vi "Compile - Rx Packet Information.vi"(8 "error in (no error)":errorcluster, 11 "Custom Device Ref in":T1 format="%.0x") -> (0 "error out":errorcluster, 1 "Rx Ref Array":T2(array[cluster]) {"VS Refs" format="%.0x"}, 2 "Rx Packet Info Array":T3[](array[typedef]) {"Endianness" items=["big-endian"=0, "little-indian"=2]}, 3 "Custom Device Ref out":T1 format="%.0x")   [LabVIEW 2016, in "UDP-Custom-Device System Explorer.lvlib"]
uses:
  UDP-Custom-Device System Explorer.lvlib
  Shared/Types/Shared - Rx.PacketInfo.ctl
  Shared/Types/Shared - Channel Data Type.ctl
  Shared/Types/Shared - Buffered.PacketInfo.ctl
  Shared/Types/Shared - Pointer Encoding.ctl
  Shared/Types/Shared - Buffer Options.ctl
  Shared/Types/Shared - Duplex Settings.ctl
  Shared/Types/Shared - New Data Options.ctl
  <vilib>/NI Veristand/Custom Device API/Custom Device Item Ref.ctl
  Shared/UDP-Custom-Device Shared.lvlib
  <vilib>/NI VeriStand/Custom Device API/Custom Device API.lvlib
  Property Accessors/Rx Channel Accessors.lvlib
  Property Accessors/Shared Packet Accessors.lvlib
  Property Accessors/Rx Packet Accessors.lvlib
  Property Accessors/Buffered Data Packet.lvlib
  Property Accessors/Rx Channel Section Accessors.lvlib
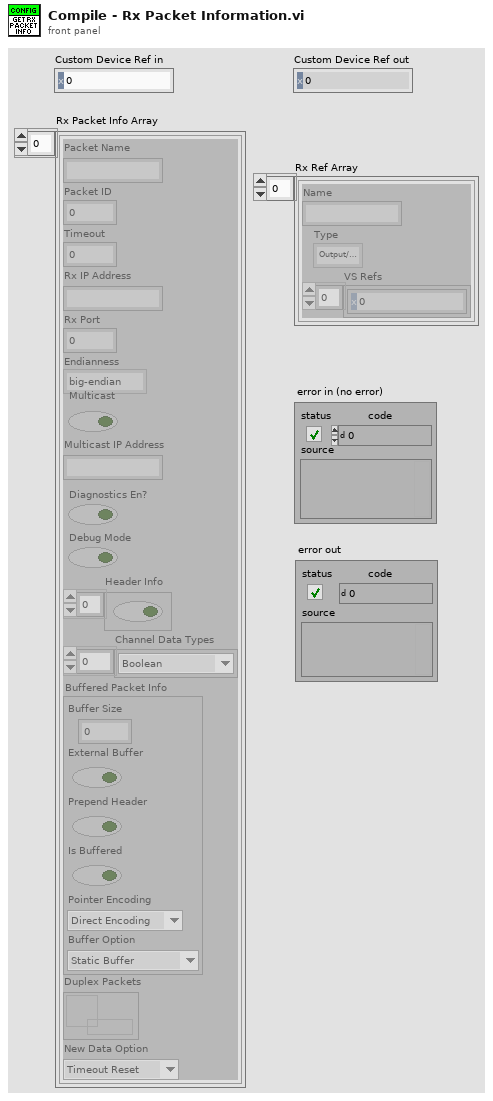
[diagram p1: front panel]
types:
  T1 = typedef "Custom Device API.lvlib/Custom Device Item Ref.ctl" = u64
  T2 = cluster{"Name":string, "Type":enum16{"Output/Write", "Input/Read", "Input/ReadWrite"}, "VS Refs":T1[]}[]
  T3 = typedef "UDP-Custom-Device Shared.lvlib/Shared - Rx.PacketInfo.ctl" = cluster{"Packet Name":string, "Packet ID":i32, "Timeout":i32, "Rx IP Address":string, "Rx Port":u16, "Endianness":u16, "Multicast":bool, "Multicast IP Address":string, "Diagnostics En?":bool, "Debug Mode":bool, "Header Info":bool[], "Channel Data Types":T4[], "Buffered Packet Info":T5, "Duplex Packets":refnum<data-value>, "New Data Option":T8}
  T4 = typedef "UDP-Custom-Device Shared.lvlib/Shared - Channel Data Type.ctl" = enum16{"Boolean", "Single", "Double", "I8", "I16", "I32", "I64", "U8", "U16", "U32", "U64"}
  T5 = typedef "UDP-Custom-Device Shared.lvlib/Shared - Buffered.PacketInfo.ctl" = cluster{"Buffer Size":i32, "External Buffer":bool, "Prepend Header":bool, "Is Buffered":bool, "Pointer Encoding":T6, "Buffer Option":T7}
  T6 = typedef "UDP-Custom-Device Shared.lvlib/Shared - Pointer Encoding.ctl" = enum16{"Direct Encoding", "Conversion Encoding"}
  T7 = typedef "UDP-Custom-Device Shared.lvlib/Shared - Buffer Options.ctl" = enum16{"Static Buffer", "Circular Buffer"}
  T8 = typedef "UDP-Custom-Device Shared.lvlib/Shared - New Data Options.ctl" = enum16{"Timeout Reset", "Counter"}
  T9 = typedef "UDP-Custom-Device System Explorer.lvlib/Packet Type.ctl" = enum16{"Transmit", "Receive", "Buffered Transmit", "Buffered Receive"}
  T10 = typedef "Custom Device API.lvlib/Custom Device Item Info.ctl" = cluster{"Name":string, "Is Channel":bool, "GUID":string, "Is Waveform":bool}
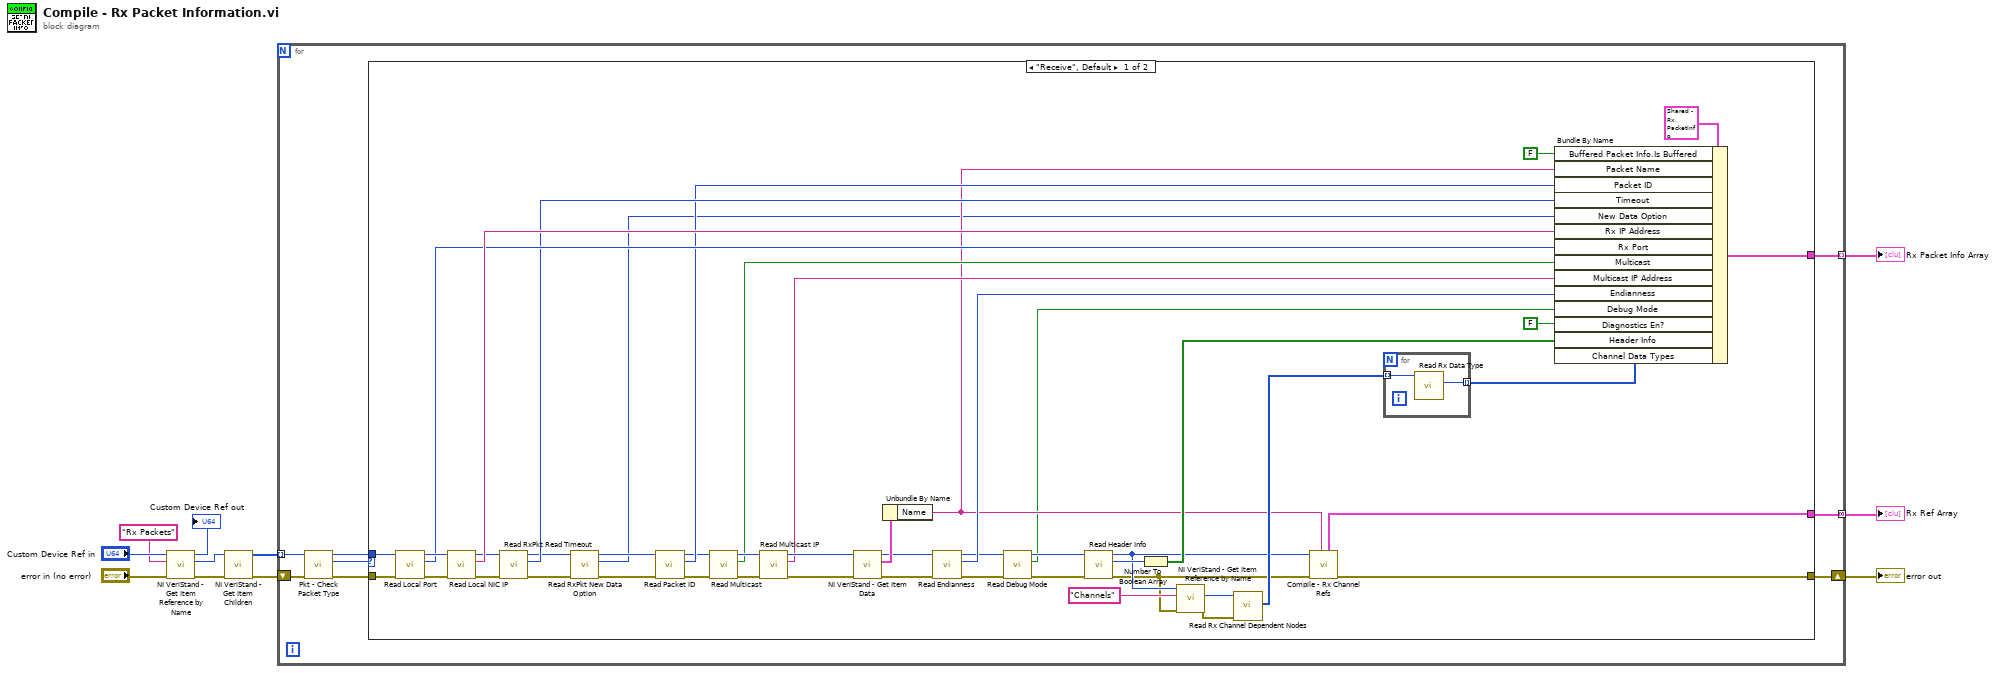
[diagram p0: block diagram]
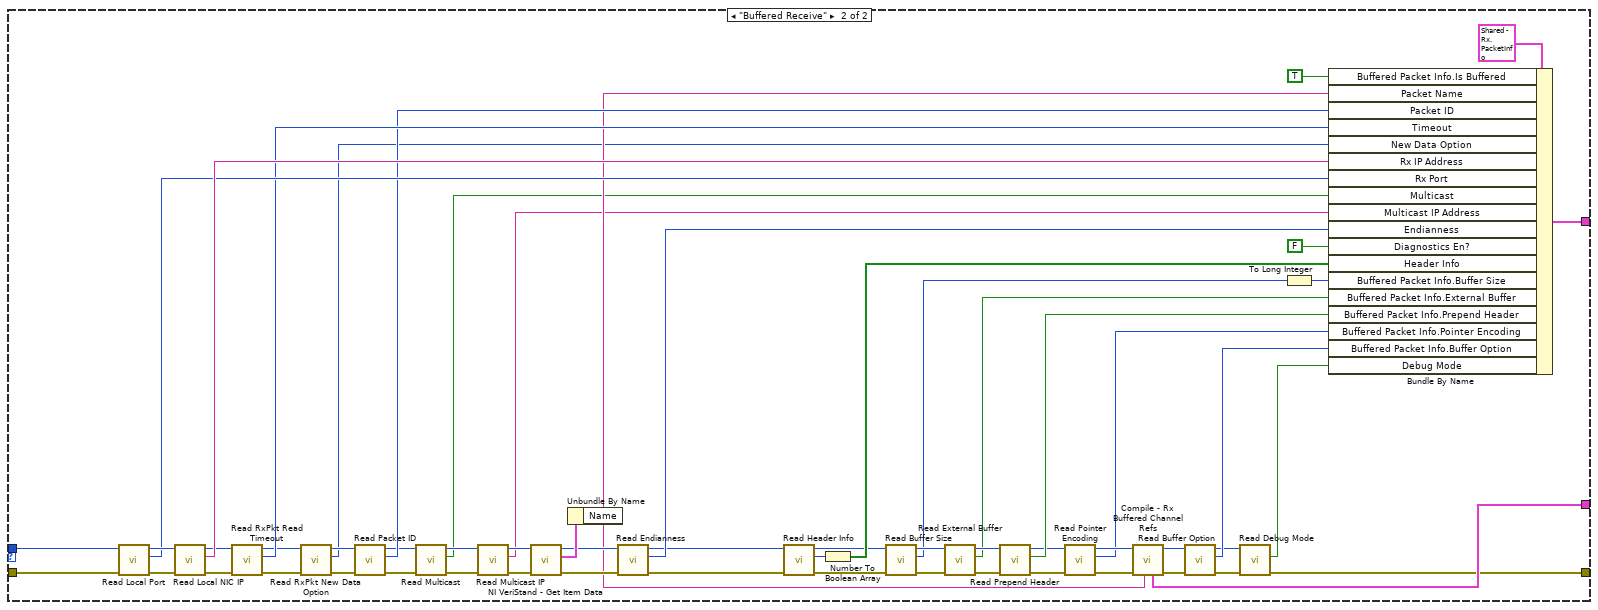
[diagram p2: hidden frame]
diagram:
  n1 = call <vilib>:"NI VeriStand - Get Item Reference by Name.vi"("error in (no error)"="error in (no error)", "Item Name"="Rx Packets", "Parent Ref in"="Custom Device Ref in") -> ("error out"=w5:errorcluster, "Item Ref"=w2:T1, "Parent Ref out"=→"Custom Device Ref out":T1)  [unwired: 5 in, 1 out]
  n2 = call <vilib>:"NI VeriStand - Get Item Children.vi"("error in (no error)"=w5, "Item Ref in"=w2) -> ("error out"=w8:errorcluster, "Child Refs"=w7:T1[])  [unwired: 6 in, 2 out]
  n3 = for {
    tunnel: w7 -> [w17] mode=indexing
    shift-right: [w18] -> w10
    shift-left: w8 -> [w15]
    tunnel: [w19] -> w9 mode=indexing
    tunnel: [w13] -> w6 mode=concatenating
    n4 = call "Pkt - Check Packet Type.vi"("error in (no error)"=w15, "Node Ptr In"=w17) -> ("error out"=w14:errorcluster, "Packet Type"=w12:T9, "Node Ptr Out"=w16:T1)  [unwired: 7 in]
    n5 = case shown="\"Receive\", Default" w12 {
      tunnel: [w66 w127] -> w19
      tunnel: [w32 w71] -> w18
      tunnel: w16 -> [w45 w110]
      tunnel: w14 -> [w44 w109]
      tunnel: [w31 w95] -> w13
      frame "Receive", Default {
        n6 = call "Read Local Port.vi"("error in (no error)"=w44, "Node Ptr"=w45) -> ("error out"=w56:errorcluster, "Port"=w57:u16, "Node Ptr out"=w59:T1)  [unwired: 7 in]
        n7 = call "Read Local NIC IP.vi"("error in (no error)"=w56, "Node Ptr"=w59) -> ("error out"=w52:errorcluster, "IP Address of Local NIC"=w58:string, "Node Ptr out"=w53:T1)  [unwired: 7 in]
        n8 = call "Read RxPkt Read Timeout.vi"("error in (no error)"=w52, "Node Ptr"=w53) -> ("error out"=w27:errorcluster, "Read Timeout"=w55:i32, "Node Ptr out"=w29:T1)  [unwired: 7 in]
        n9 = call "Read RxPkt New Data Option.vi"("error in (no error)"=w27, "Node Ptr"=w29) -> ("error out"=w26:errorcluster, "New Data Option"=w25:T8, "Node Ptr out"=w28:T1)  [unwired: 7 in]
        n10 = call "Read Packet ID.vi"("error in (no error)"=w26, "Node Ptr"=w28) -> ("error out"=w36:errorcluster, "Packet ID"=w54:i32, "Node Ptr out"=w35:T1)  [unwired: 7 in]
        n11 = call "Read Multicast.vi"("error in (no error)"=w36, "Node Ptr"=w35) -> ("error out"=w41:errorcluster, "Multicast"=w38:bool, "Node Ptr out"=w42:T1)  [unwired: 7 in]
        n12 = call "Read Multicast IP.vi"("error in (no error)"=w41, "Node Ptr"=w42) -> ("error out"=w39:errorcluster, "Multicast IP Address"=w37:string, "Node Ptr out"=w40:T1)  [unwired: 7 in]
        n13 = call <vilib>:"NI VeriStand - Get Item Data.vi"("error in (no error)"=w39, "Item Ref in"=w40) -> ("error out"=w48:errorcluster, "Item Info"=w51:T10, "Item Ref out"=w49:T1)  [unwired: 6 in, 1 out]
        n14 = Unbundle By Name(w51) -> ("Name"=w30:string)
        n15 = call "Read Endianness.vi"("error in (no error)"=w48, "Node Ptr"=w49) -> ("error out"=w22:errorcluster, "Endianness"=w47:u16, "Node Ptr out"=w24:T1)  [unwired: 7 in]
        n16 = call "Read Debug Mode.vi"("error in (no error)"=w22, "Node Ptr"=w24) -> ("error out"=w21:errorcluster, "Debug Mode"=w20:bool, "Node Ptr out"=w23:T1)  [unwired: 7 in]
        n17 = call "Read Header Info.vi"("error in (no error)"=w21, "Node Ptr"=w23) -> ("error out"=w33:errorcluster, "Header Info"=w46:u32, "Node Ptr out"=w34:T1)  [unwired: 7 in]
        n18 = Number To Boolean Array(number=w46) -> (Boolean array=w65:bool[])
        n19 = call <vilib>:"NI VeriStand - Get Item Reference by Name.vi"("error in (no error)"=w33, "Item Name"="Channels" ("Section Name"), "Parent Ref in"=w34) -> ("error out"=w62:errorcluster, "Item Ref"=w63:T1)  [unwired: 5 in, 2 out]
        n20 = call "Read Rx Channel Dependent Nodes.vi"("error in (no error)"=w62, "Node Ptr"=w63) -> ("Dependent Node Refs"=w61:T1[])  [unwired: 7 in, 2 out]
        n21 = call "Compile - Rx Channel Refs.vi"("Packet Name"=w30, "error in (no error)"=w33, "Item Ref in"=w34) -> ("error out"=w32:errorcluster, "Rx Ref Array"=w31:T2)  [unwired: 6 in, 1 out]
        n22 = for {
          tunnel: w61 -> [w69] mode=indexing
          tunnel: [w68] -> w60 mode=indexing
          n23 = call "Read Rx Data Type.vi"("Node Ptr"=w69) -> ("Data Type"=w68:T4)  [unwired: 8 in, 2 out]
        }
        n24 = Bundle By Name(cluster=T3 {"Packet Name"="", "Packet ID"=0, "Timeout"=0, "Rx IP Address"="", "Rx Port"=0, "Endianness"=0, "Multicast"=FALSE, "Multicast IP Address"="", "Diagnostics En?"=FALSE, "Debug Mode"=FALSE, "Header Info"=[], "Channel Data Types"=[], "Buffered Packet Info"={"Buffer Size"=0, "External Buffer"=FALSE, "Prepend Header"=FALSE, "Is Buffered"=FALSE, "Pointer Encoding"=enum."Direct Encoding", "Buffer Option"=enum."Static Buffer"}, "Duplex Packets"=refnum, "New Data Option"=enum."Timeout Reset"} ("Packet Info"), "Buffered Packet Info.Is Buffered"=FALSE, "Packet Name"=w30, "Packet ID"=w54, "Timeout"=w55, "New Data Option"=w25, "Rx IP Address"=w58, "Rx Port"=w57, "Multicast"=w38, "Multicast IP Address"=w37, "Endianness"=w47, "Debug Mode"=w20, "Diagnostics En?"=FALSE, "Header Info"=w65, "Channel Data Types"=w60) -> (w66:T3)
      }
      frame "Buffered Receive" {
        n25 = call "Read Local Port.vi"("error in (no error)"=w109, "Node Ptr"=w110) -> ("error out"=w123:errorcluster, "Port"=w124:u16, "Node Ptr out"=w126:T1)  [unwired: 7 in]
        n26 = call "Read Local NIC IP.vi"("error in (no error)"=w123, "Node Ptr"=w126) -> ("error out"=w119:errorcluster, "IP Address of Local NIC"=w125:string, "Node Ptr out"=w120:T1)  [unwired: 7 in]
        n27 = call "Read RxPkt Read Timeout.vi"("error in (no error)"=w119, "Node Ptr"=w120) -> ("error out"=w81:errorcluster, "Read Timeout"=w122:i32, "Node Ptr out"=w79:T1)  [unwired: 7 in]
        n28 = call "Read RxPkt New Data Option.vi"("error in (no error)"=w81, "Node Ptr"=w79) -> ("error out"=w80:errorcluster, "New Data Option"=w77:T8, "Node Ptr out"=w78:T1)  [unwired: 7 in]
        n29 = call "Read Packet ID.vi"("error in (no error)"=w80, "Node Ptr"=w78) -> ("error out"=w87:errorcluster, "Packet ID"=w121:i32, "Node Ptr out"=w88:T1)  [unwired: 7 in]
        n30 = call "Read Multicast.vi"("error in (no error)"=w87, "Node Ptr"=w88) -> ("error out"=w93:errorcluster, "Multicast"=w90:bool, "Node Ptr out"=w94:T1)  [unwired: 7 in]
        n31 = call "Read Multicast IP.vi"("error in (no error)"=w93, "Node Ptr"=w94) -> ("error out"=w92:errorcluster, "Multicast IP Address"=w89:string, "Node Ptr out"=w91:T1)  [unwired: 7 in]
        n32 = call <vilib>:"NI VeriStand - Get Item Data.vi"("error in (no error)"=w92, "Item Ref in"=w91) -> ("error out"=w115:errorcluster, "Item Info"=w118:T10, "Item Ref out"=w116:T1)  [unwired: 6 in, 1 out]
        n33 = Unbundle By Name(w118) -> ("Name"=w96:string)
        n34 = call "Read Endianness.vi"("error in (no error)"=w115, "Node Ptr"=w116) -> ("error out"=w112:errorcluster, "Endianness"=w114:u16, "Node Ptr out"=w113:T1)  [unwired: 7 in]
        n35 = call "Read Header Info.vi"("error in (no error)"=w112, "Node Ptr"=w113) -> ("error out"=w98:errorcluster, "Header Info"=w111:u32, "Node Ptr out"=w99:T1)  [unwired: 7 in]
        n36 = Number To Boolean Array(number=w111) -> (Boolean array=w107:bool[])
        n37 = call "Read Buffer Size.vi"("error in (no error)"=w98, "Node Ptr"=w99) -> ("error out"=w106:errorcluster, "Buffer Size"=w103:u32, "Node Ptr out"=w104:T1)  [unwired: 7 in]
        n38 = call "Read External Buffer.vi"("error in (no error)"=w106, "Node Ptr"=w104) -> ("error out"=w105:errorcluster, "External Buffer"=w97:bool, "Node Ptr out"=w102:T1)  [unwired: 7 in]
        n39 = call "Read Prepend Header.vi"("error in (no error)"=w105, "Node Ptr"=w102) -> ("error out"=w84:errorcluster, "Prepend Header"=w101:bool, "Node Ptr out"=w86:T1)  [unwired: 7 in]
        n40 = call "Read Pointer Encoding.vi"("error in (no error)"=w84, "Node Ptr"=w86) -> ("error out"=w83:errorcluster, "Pointer Encoding"=w82:T6, "Node Ptr out"=w85:T1)  [unwired: 7 in]
        n41 = call "Compile - Rx Buffered Channel Refs.vi"("Packet Name"=w96, "error in (no error)"=w83, "Item Ref in"=w85) -> ("error out"=w75:errorcluster, "Item Ref out"=w76:T1, "Rx Ref Array"=w95:T2)  [unwired: 6 in]
        n42 = call "Read Buffer Option.vi"("error in (no error)"=w75, "Node Ptr"=w76) -> ("error out"=w72:errorcluster, "Buffer Option"=w74:T7, "Node Ptr out"=w73:T1)  [unwired: 7 in]
        n43 = call "Read Debug Mode.vi"("error in (no error)"=w72, "Node Ptr"=w73) -> ("error out"=w71:errorcluster, "Debug Mode"=w70:bool)  [unwired: 7 in, 1 out]
        n44 = To Long Integer(number=w103) -> (32bit integer=w100:i32)
        n45 = Bundle By Name(cluster=T3 {"Packet Name"="", "Packet ID"=0, "Timeout"=0, "Rx IP Address"="", "Rx Port"=0, "Endianness"=0, "Multicast"=FALSE, "Multicast IP Address"="", "Diagnostics En?"=FALSE, "Debug Mode"=FALSE, "Header Info"=[], "Channel Data Types"=[], "Buffered Packet Info"={"Buffer Size"=0, "External Buffer"=FALSE, "Prepend Header"=FALSE, "Is Buffered"=FALSE, "Pointer Encoding"=enum."Direct Encoding", "Buffer Option"=enum."Static Buffer"}, "Duplex Packets"=refnum, "New Data Option"=enum."Timeout Reset"} ("Packet Info"), "Buffered Packet Info.Is Buffered"=TRUE, "Packet Name"=w96, "Packet ID"=w121, "Timeout"=w122, "New Data Option"=w77, "Rx IP Address"=w125, "Rx Port"=w124, "Multicast"=w90, "Multicast IP Address"=w89, "Endianness"=w114, "Diagnostics En?"=FALSE, "Header Info"=w107, "Buffered Packet Info.Buffer Size"=w100, "Buffered Packet Info.External Buffer"=w97, "Buffered Packet Info.Prepend Header"=w101, "Buffered Packet Info.Pointer Encoding"=w82, "Buffered Packet Info.Buffer Option"=w74, "Debug Mode"=w70) -> (w127:T3)
      }
    }
  }
  "Rx Packet Info Array" <- w9
  "error out" <- w10
  "Rx Ref Array" <- w6
